vi "Loop Timeout.vi"(1 "App in":refnum<class "App.lvclass">) -> (0 "Timeout":i32)   [LabVIEW 2020, in "AR Example.lvlib" / "App.lvclass"]
uses:
  App.lvclass
  App.lvclass/App.ctl
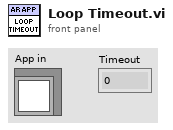
[diagram p1: front panel]
types:
  T1 = typedef "AR Example.lvlib/App.lvclass/Timeout Action.ctl" = enum16{"None", "Setup Camera Action", "Camera Calibration Action"}
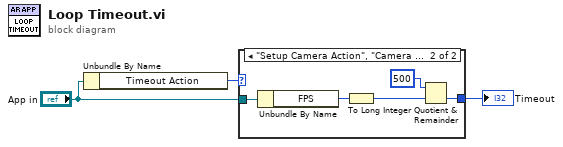
[diagram p0: block diagram]
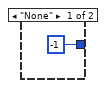
[diagram p2: hidden frame]
diagram:
  n1 = Unbundle By Name("App in") -> ("Timeout Action"=w3:T1)
  n2 = case shown="\"Setup Camera Action\", \"Camera Calibration Action\"" w3 {
    tunnel: [-1 w5] -> w2
    tunnel: "App in" -> [_ w9]
    frame "None" {
    }
    frame "Setup Camera Action", "Camera Calibration Action" {
      n3 = Unbundle By Name(w9) -> ("FPS"=w7:u8)
      n4 = To Long Integer(number=w7) -> (32bit integer=w6:i32)
      n5 = Quotient & Remainder(x=500, y=w6) -> (floor(x/y)=w5:i32)  [unwired: 1 out]
    }
  }
  "Timeout" <- w2
